vi "TCP_in_MSG.vi"(10 "msg i":string) -> (1 "rsp":u32, 2 "msg o":string, 3 "cmd":u32)   [LabVIEW 2020, in "FINS TCP.lvlib"]
uses:
  FINS TCP.lvlib
panel:
  out "length 2":i32
  out "length":u32
  out "FINS":string
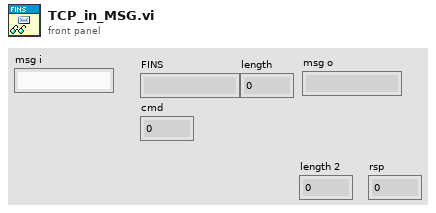
[diagram p1: front panel]
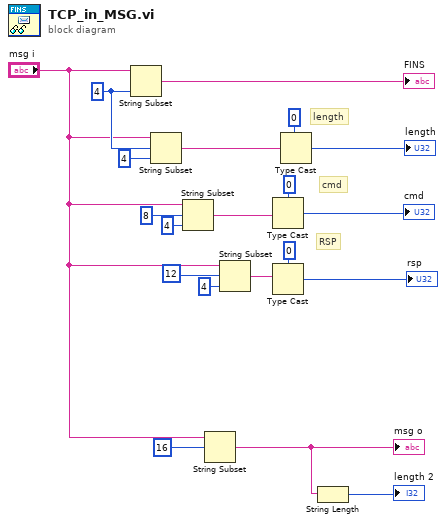
[diagram p0: block diagram]
diagram:
  w14 = 4 ("length (rest)")
  # "RSP"
  # "cmd"
  # "length"
  n1 = String Subset(string="msg i", length (rest)=w14) -> (substring=→"FINS":string)  [unwired: 1 in]
  n2 = String Subset(string="msg i", offset (0)=w14, length (rest)=4 ("length (rest)")) -> (substring=w16:string)
  n3 = String Subset(string="msg i", offset (0)=8 ("length (rest)"), length (rest)=4 ("length (rest)")) -> (substring=w10:string)
  n4 = String Subset(string="msg i", offset (0)=16 ("length (rest)")) -> (substring=w5:string)  [unwired: 1 in]
  "msg o" <- w5
  n5 = String Subset(string="msg i", offset (0)=12 ("length (rest)"), length (rest)=4 ("length (rest)")) -> (substring=w2:string)
  n6 = Type Cast(type=u32 0 ("length"), x=w10) -> (*(type *) &x=→"cmd":u32)
  n7 = Type Cast(type=u32 0 ("length"), x=w2) -> (*(type *) &x=→"rsp":u32)
  n8 = Type Cast(type=u32 0 ("length"), x=w16) -> (*(type *) &x=→"length":u32)
  n9 = String Length(string=w5) -> (length=→"length 2":i32)
